vi "constructModuleLibrary.vi"(8 "error in (no error)":errorcluster, 10 "targetBasePath":path, 11 "Module in":refnum<class "Module.lvclass">) -> (0 "error out":errorcluster, 3 "Module out":refnum<class "Module.lvclass">)   [LabVIEW 2016, in "Module.lvclass"]
uses:
  Module.lvclass
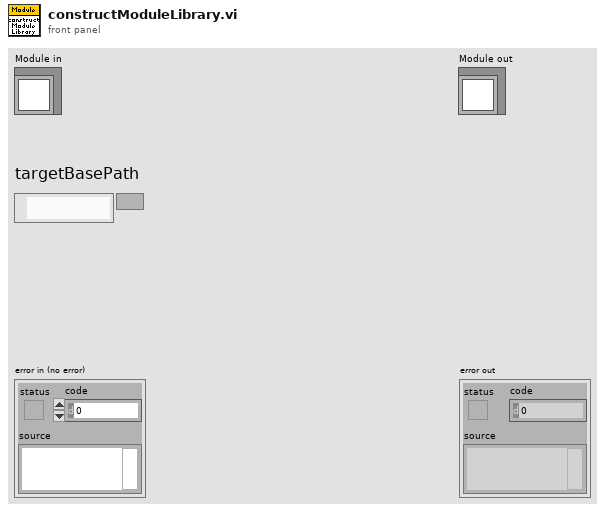
[diagram p1: front panel]
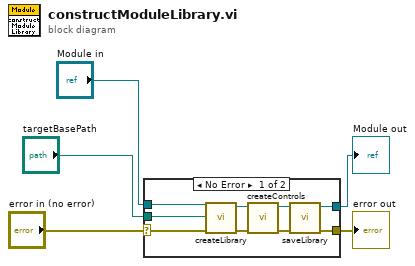
[diagram p0: block diagram]
diagram:
  n1 = case shown="No Error" "error in (no error)" {
    selector: "error in (no error)" -> [w6 w16]
    tunnel: [w9 w16] -> w4
    tunnel: [w11 w15] -> w2
    tunnel: "Module in" -> [w8 w15]
    tunnel: "targetBasePath" -> [w7 _]
    frame No Error {
      n2 = call "createLibrary.vi"("error in (no error)"=w6, "directoryPath"=w7, "Module in"=w8) -> ("error out"=w13:errorcluster, "Module out"=w14:refnum<class "Module.lvclass">)  [unwired: 7 in]
      n3 = call "createControls.vi"("error in (no error)"=w13, "Module in"=w14) -> ("error out"=w10:errorcluster, "Module out"=w12:refnum<class "Module.lvclass">)  [unwired: 8 in]
      n4 = call "saveLibrary.vi"("error in (no error)"=w10, "Module in"=w12) -> ("error out"=w9:errorcluster, "Module out"=w11:refnum<class "Module.lvclass">)  [unwired: 8 in]
    }
    frame Error {
    }
  }
  "error out" <- w4
  "Module out" <- w2
